vi "File.Remove Name Extension.vi"(3 "File Name":string) -> (0 "Ext":string, 1 "Name Less Ext":string)   [LabVIEW 2024, in "EQMF.lvlib" / "File Utils.lvlib"]
doc: "This VI removes the extension from a file name.\n\nEXAMPLE:\n Input file name \"ABCD.txt\" will output \"ABCD\""
uses:
  File Utils.lvlib
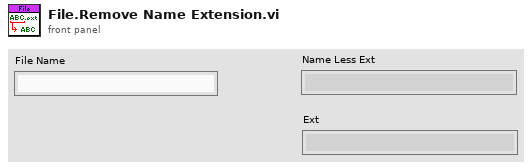
[diagram p1: front panel]
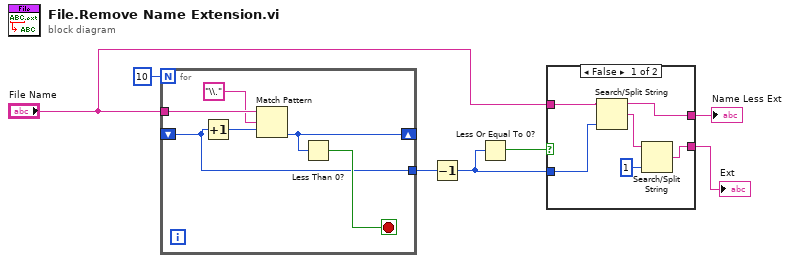
[diagram p0: block diagram]
diagram:
  n1 = for {
    N: 10 -> [_]
    shift-right: [w12] -> _
    shift-left: _ -> [w8]
    tunnel: "File Name" -> [w13]
    tunnel: [w8] -> w4
    stop <- w10 stop-if-true
    n2 = Increment(x=w8) -> (x+1=w11:i32)
    n3 = Match Pattern(string=w13, regular expression="\\.", offset (0)=w11) -> (offset past match=w12:i32)  [unwired: 3 out]
    n4 = Less Than 0?(x=w12) -> (x < 0?=w10:bool)
  }
  n5 = Decrement(x=w4) -> (x-1=w3:i32)
  n6 = Less Or Equal To 0?(x=w3) -> (x <= 0?=w2:bool)
  n7 = case shown="False" w2 {
    tunnel: "File Name" -> [w19 w20]
    tunnel: [w17 w20] -> w6
    tunnel: w3 -> [w18 _]
    tunnel: [w14 _] -> w1
    frame False {
      n8 = Search/Split String(string=w19, offset (0)=w18) -> (substring before match=w17:string, match + rest of string=w16:string)  [unwired: 1 in, 1 out]
      n9 = Search/Split String(string=w16, offset (0)=1) -> (match + rest of string=w14:string)  [unwired: 1 in, 2 out]
    }
    frame True {
    }
  }
  "Name Less Ext" <- w6
  "Ext" <- w1
